vi "Init.vi"(8 "error in (no error)":errorcluster, 11 "Kasli Wrapper in":refnum<class "Kasli Wrapper 2.0.lvclass">) -> (0 "error out":errorcluster, 3 "Kasli Wrapper out":refnum<class "Kasli Wrapper 2.0.lvclass">)   [LabVIEW 2020, in "Kasli Wrapper 2.0.lvlib" / "Kasli Wrapper 2.0.lvclass"]
uses:
  Kasli Wrapper 2.0.lvclass
  Kasli Wrapper 2.0 Consumer Case Selector.ctl
  Kasli Wrapper 2.0.lvclass/Kasli Wrapper 2.0.ctl
  TALOS/TALOS_PPL.lvlibp/Father of all uServices/Father of all uServices/Father of all uServices.lvclass
  TALOS/TALOS_PPL.lvlibp/Classes/Log/Log.lvclass
  TALOS/TALOS_PPL.lvlibp
  C:/LabVIEW Code/aegis-labview-code/TALOS/TALOS_PPL.lvlibp/Father of all uServices/Father of all uServices/Father of all uServices.lvclass
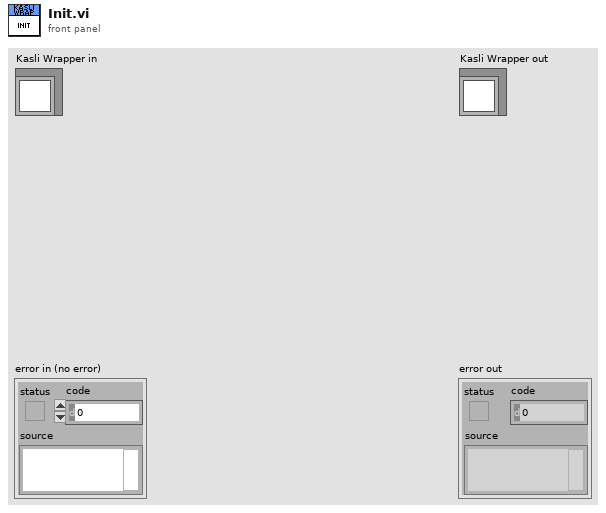
[diagram p1: front panel]
types:
  T1 = typedef "Kasli Wrapper 2.0.lvlib/Kasli Wrapper 2.0.lvclass/Kasli Wrapper 2.0 Consumer Case Selector.ctl" = enum16{"Init", "Submit Script", "Restart Master", "Master StdOut", "Master StdErr", "Client StdOut", "Client StdErr", "Start Logging", "Stop Logging", "Terminate Script", "Close", "Master ProcessExit"}
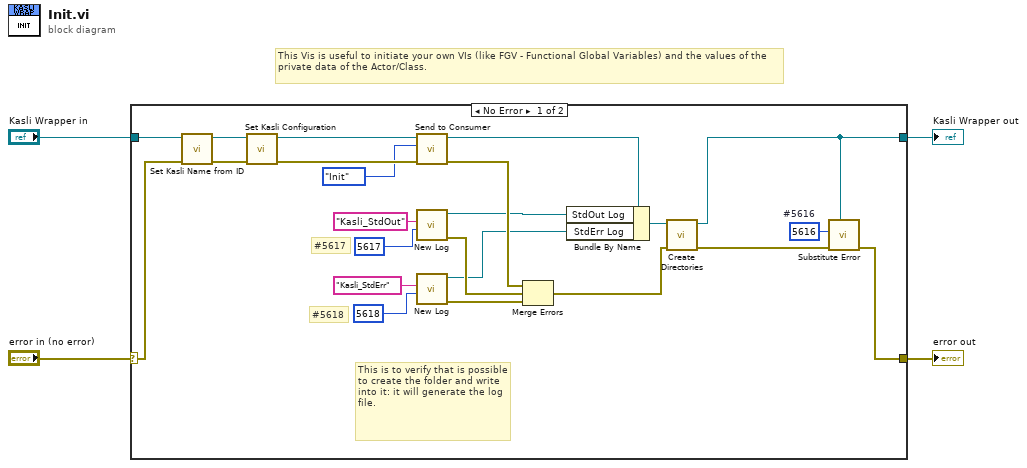
[diagram p0: block diagram]
diagram:
  # "This Vis is useful to initiate your own VIs (like FGV - Functional Global Variables) and the values of the private data of the Actor/Class."
  n1 = case shown="No Error" "error in (no error)" {
    selector: "error in (no error)" -> [w25 w28]
    tunnel: "Kasli Wrapper in" -> [w26 w29]
    tunnel: [w23 w29] -> w4
    tunnel: [w24 w28] -> w3
    frame No Error {
      w6 = 5616  # #5616
      # "#5618"
      # "#5617"
      # "This is to verify that is possible to create the folder and write into it: it will generate the log file."
      n2 = call-dynamic "Set Kasli Name from ID.vi"("error in (no error)"=w25, "Kasli Wrapper 2.0 in"=w26) -> ("error out"=w10:errorcluster, "Kasli Wrapper 2.0 out"=w11:refnum<class "Kasli Wrapper 2.0.lvclass">)  [unwired: 6 in, 2 out]
      n3 = call-dynamic "Set Kasli Configuration.vi"("error in (no error)"=w10, "Kasli Wrapper 2.0 in"=w11) -> ("error out"=w8:errorcluster, "Kasli Wrapper 2.0 out"=w9:refnum<class "Kasli Wrapper 2.0.lvclass">)  [unwired: 8 in]
      n4 = call "Send to Consumer.vi"("error in (no error)"=w8, "Case ID"=Kasli_Wrapper_2.0_Consumer_Case_Selector."Init" ("Kasli Wrapper 2 Consumer Case Selector"), "uService Template in"=w9) -> ("error out"=w27:errorcluster, "uService Template out"=w14:refnum<class "Kasli Wrapper 2.0.lvclass">)  [unwired: 7 in]
      n5 = call "New Log.vi"("Specific Error Code"=5617, "Name"="Kasli_StdOut") -> ("error out"=w18:errorcluster, "Log out"=w16:refnum<class "Log.lvclass">)  [unwired: 8 in]
      n6 = call "New Log.vi"("Specific Error Code"=5618, "Name"="Kasli_StdErr") -> ("error out"=w17:errorcluster, "Log out"=w15:refnum<class "Log.lvclass">)  [unwired: 8 in]
      n7 = Merge Errors(w27, w18, w17) -> (w13:errorcluster)
      n8 = Bundle By Name(cluster=w14, "StdOut Log"=w16, "StdErr Log"=w15) -> (w12:refnum<class "Kasli Wrapper 2.0.lvclass">)
      n9 = call-dynamic "Create Directories.vi"("error in (no error)"=w13, "Kasli Wrapper 2.0 in"=w12) -> ("error out"=w7:errorcluster, "Kasli Wrapper 2.0 out"=w23:refnum<class "Kasli Wrapper 2.0.lvclass">)  [unwired: 8 in]
      n10 = call "Substitute Error.vi"("LabVIEW Object"=w23, "error in (no error)"=w7, "Error Code"=w6) -> ("error out"=w24:errorcluster)  [unwired: 8 in]
    }
    frame Error {
    }
  }
  "error out" <- w3
  "Kasli Wrapper out" <- w4
